vi "Change_Status_In_Case_Best_101-111-1.vi"(4 "[IN] Current Status":i16, 5 "error IN":errorcluster, 6 "[IN] Track group":T1, 7 "[IN] Index of track with\nproblem displacement":i32, 8 "[IN]Index of problem dis\nplacement inside track":i32) -> (0 "error OUT":errorcluster, 3 "[OUT] Status of point after 101":i16)   [LabVIEW 2013]
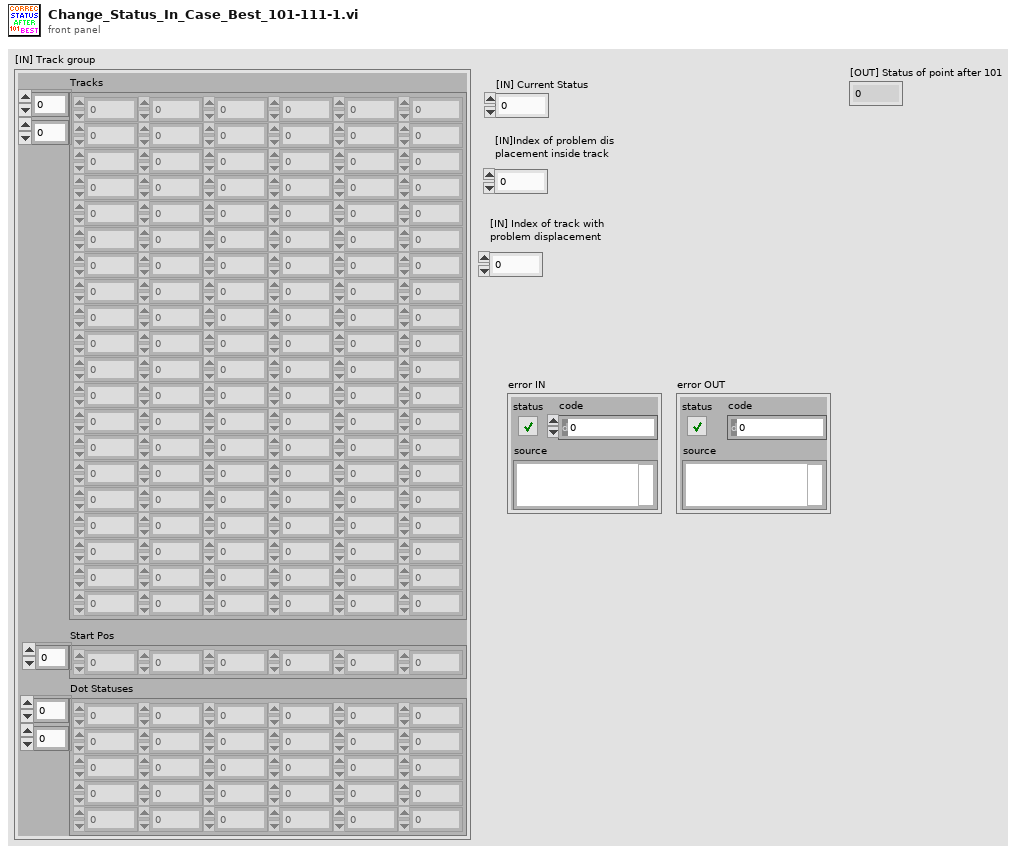
[diagram p1: front panel]
types:
  T1 = cluster{"Tracks":dbl[][], "Start Pos":i32[], "Dot Statuses":i16[][]}
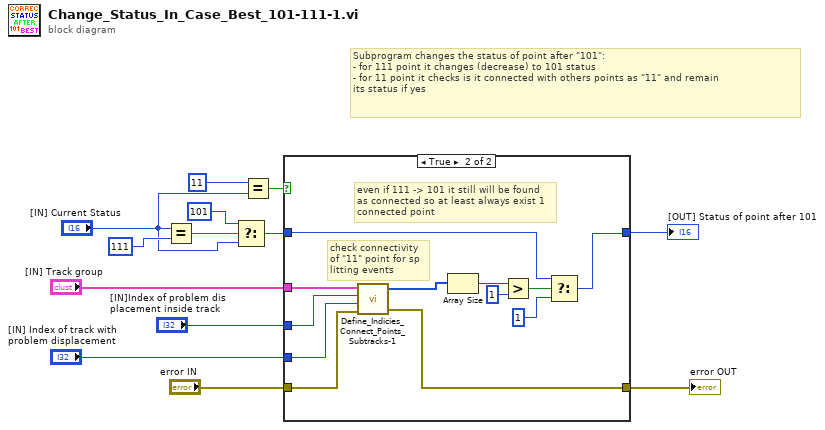
[diagram p0: block diagram]
diagram:
  # "Subprogram changes the status of point after \"101\":\n- for 111 point it changes (decrease) to 101 status\n- for 11 point it checks is it connected with others points as \"11\" and remain \nits status if yes"
  n1 = Equal?(x="[IN] Current Status", y=i16 111) -> (x = y?=w12:bool)
  n2 = Select(t=i16 101, s=w12, f="[IN] Current Status") -> (s? t:f=w7:i16)
  n3 = Equal?(x=i16 11, y="[IN] Current Status") -> (x = y?=w8:bool)
  n4 = case shown="True" w8 {
    tunnel: w7 -> [w15 w21]
    tunnel: "[IN] Track group" -> [_ w26]
    tunnel: "[IN]Index of problem dis\nplacement inside track" -> [_ w25]
    tunnel: "[IN] Index of track with\nproblem displacement" -> [_ w24]
    tunnel: "error IN" -> [w14 w23]
    tunnel: [w15 w19] -> w1
    tunnel: [w14 w18] -> w2
    frame False {
    }
    frame True {
      # "even if 111 -> 101 it still will be found\nas connected so at least always exist 1 \nconnected point"
      # "check connectivity \nof \"11\" point for sp\nlitting events"
      n5 = call "Define_Indicies_Connect_Points_Subtracks-1.vi"("error IN"=w23, "[IN] Index of track with\n(problem displacement)"=w24, "[IN] Index of problem\ndisplacement inside track"=w25, "[IN] Track group"=w26) -> ("error OUT"=w18:errorcluster, "[OUT] Index of connected\ntracks with problem dot"=w27:i32[])  [unwired: 1 out]
      n6 = Array Size(array=w27) -> (size(s)=w17:i32)
      n7 = Greater?(x=w17, y=1) -> (0:w22:bool)
      n8 = Select(t=w21, s=w22, f=i16 1) -> (s? t:f=w19:i16)
    }
  }
  "error OUT" <- w2
  "[OUT] Status of point after 101" <- w1
